vi "Train Track SVM.vi"(8 "error in (no error)":errorcluster, 9 "Classifier File":path=path "C:/Users/Andrew/Documents/Apatite to Zircon Code/Track Finding/TrackClassifier.svm", 10 "Non-track Data File":path=path "C:/Users/Andrew/Documents/Apatite to Zircon Code/Track Finding/Non-track Data.csv", 11 "Track Data File":path=path "C:/Users/Andrew/Documents/Apatite to Zircon Code/Track Finding/Track Data.csv") -> (0 "error out":errorcluster, 1 "Class Predictive Value":dbl[](array[numeric]) format="%.2f", 2 "Classification Distribution":i32[][](array[numeric]), 3 "Accuracy":sgl format="%.2f")   [LabVIEW 2013]
uses:
  <vilib>/vision/Classification.llb/IMAQ SVM Kernel Options.ctl
  <vilib>/vision/Classification.llb/IMAQ SVM Model Options.ctl
  <vilib>/Utility/file.llb/Read From Spreadsheet File (DBL).vi
  <vilib>/vision/NI_Vision_Development_Module.lvlib
panel:
  in  "Model Options":T1={"SVM Model"=enum."C-SVC", "Tolerance"=0.001, "Max. Iteration"=100000, "Nu"=0.1, "Shrinking"=TRUE, "Cost"=1.0, "Weighted Cost"=[]}
  in  "Kernel Options":T2={"Kernel"=enum."Linear", "Degree"=3, "Gamma"=1.0, "Coefficient"=0.0, "Sigma"=1.0, "Cache(MB)"=10.0}
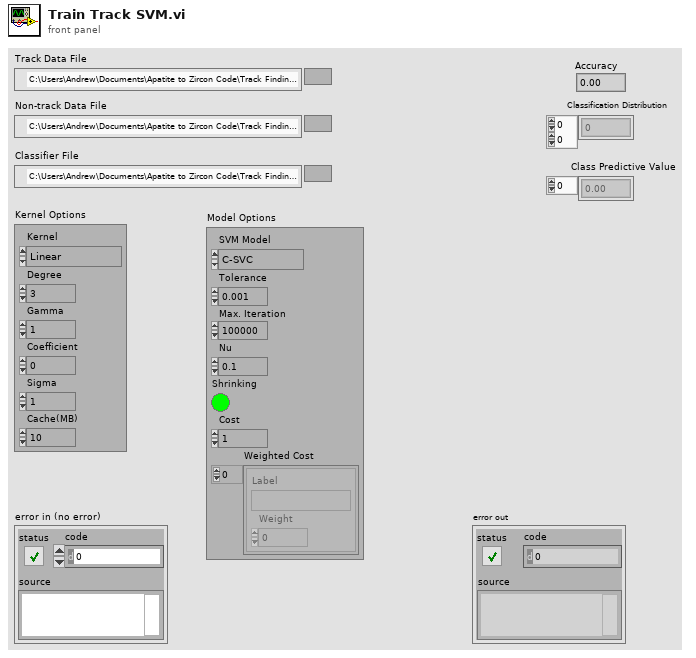
[diagram p1: front panel]
types:
  T1 = typedef "IMAQ SVM Model Options.ctl" = cluster{"SVM Model":enum32{"C-SVC", "nu-SVC", "One Class"}, "Tolerance":dbl, "Max. Iteration":i32, "Nu":dbl, "Shrinking":bool, "Cost":dbl, "Weighted Cost":cluster{"Label":string, "Weight":dbl}[]}
  T2 = typedef "IMAQ SVM Kernel Options.ctl" = cluster{"Kernel":enum32{"Linear", "Polynomial", "Gaussian", "RBF"}, "Degree":i32, "Gamma":dbl, "Coefficient":dbl, "Sigma":dbl, "Cache(MB)":dbl}
  T3 = typedef "Image Type" = u32
  T4 = typedef "IMAQ Image.ctl" = refnum<image>
  T5 = typedef "IMAQ Classifier Session.ctl" = refnum<k1>
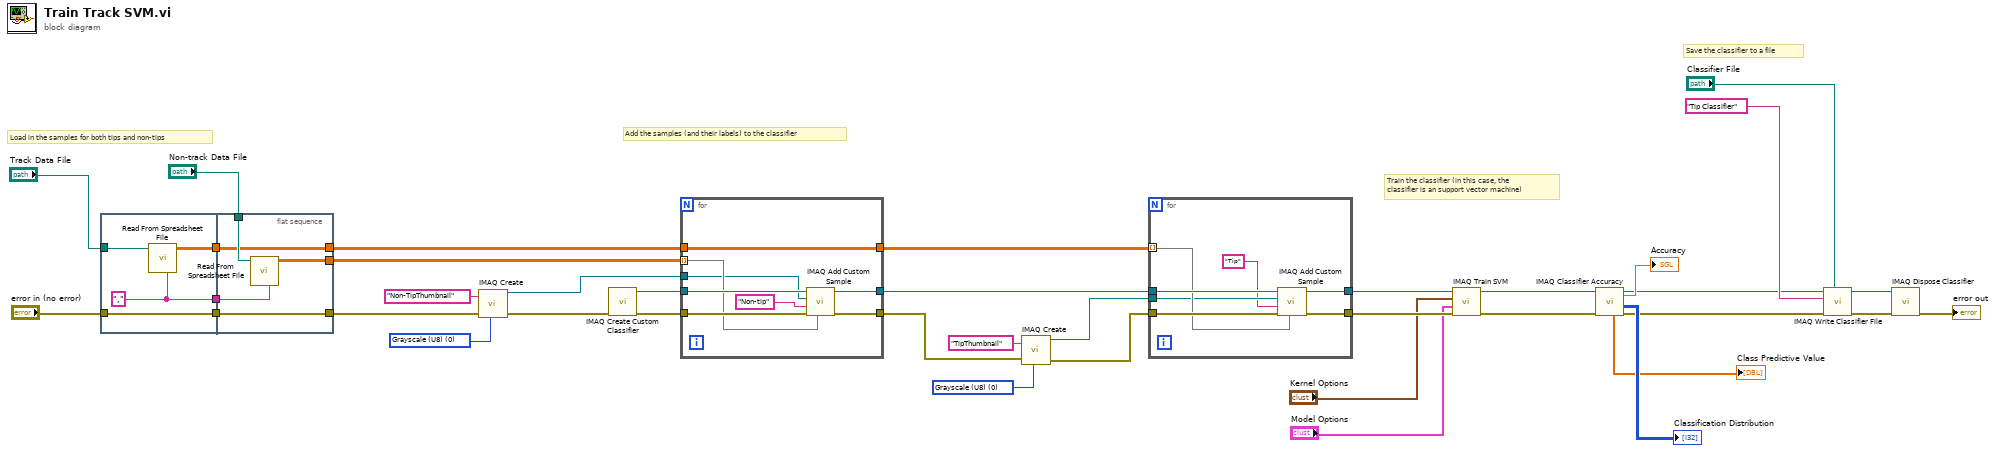
[diagram p0: block diagram]
diagram:
  w27 = T3 0 items=["Grayscale (U8)", "Grayscale (I16)", "Grayscale (SGL)", "Complex (CSG)", "RGB (U32)", "HSL (U32)", "RGB (U64)", "Grayscale (U16)"] ("Image Type")
  w29 = T3 0 items=["Grayscale (U8)", "Grayscale (I16)", "Grayscale (SGL)", "Complex (CSG)", "RGB (U32)", "HSL (U32)", "RGB (U64)", "Grayscale (U16)"] ("Image Type")
  # "Save the classifier to a file"
  # "Train the classifier (in this case, the \nclassifier is an support vector machine)"
  # "Add the samples (and their labels) to the classifier"
  # "Load in the samples for both tips and non-tips"
  n1 = flat-sequence {
    tunnel: "Track Data File" -> [w42]
    tunnel: "error in (no error)" -> [w41]
    tunnel: [w41] -> w36
    tunnel: [w40] -> w34
    tunnel: [w39] -> w22
    tunnel: [w47] -> w25
    tunnel: w36 -> [w47]
    tunnel: "Non-track Data File" -> [w46]
    tunnel: [w45] -> w20
    tunnel: w34 -> [w44]
    tunnel: [w44] -> w21
    tunnel: w22 -> [w43]
    frame #0 {
      w39 = "," ("delimiter (\\t)")
      n2 = call-poly <vilib>:"Read From Spreadsheet File.vi"("delimiter (\\t)"=w39, "file path (dialog if empty)"=w42) -> ("all rows"=w40:dbl[][])  [unwired: 5 in, 4 out]
    }
    frame #1 {
      n3 = call-poly <vilib>:"Read From Spreadsheet File.vi"("delimiter (\\t)"=w43, "file path (dialog if empty)"=w46) -> ("all rows"=w45:dbl[][])  [unwired: 5 in, 4 out]
    }
  }
  n4 = call "IMAQ Create"("Image Name"="Non-TipThumbnail", "Image Type"=w27, "error in (no error)"=w25) -> ("New Image"=w19:T4, "error out"=w18:errorcluster)  [unwired: 2 in]
  n5 = call "IMAQ Create Custom Classifier"("error in (no error)"=w18) -> ("error out"=w32:errorcluster, "Classifier Session"=w33:T5)  [unwired: 9 in]
  n6 = for {
    tunnel: w20 -> [w53] mode=indexing
    tunnel: w33 -> [w54]
    tunnel: w32 -> [w55]
    tunnel: [w52] -> w30
    tunnel: [w51] -> w24
    tunnel: w21 -> [w50]
    tunnel: [w50] -> w31
    tunnel: w19 -> [w48]
    n7 = call "IMAQ Add Custom Sample"("Feature Vector"=w53, "error in (no error)"=w55, "Class"="Non-tip", "Image"=w48, "Classifier Session"=w54) -> ("error out"=w51:errorcluster, "Classifier Session (dup)"=w52:T5)  [unwired: 5 in]
  }
  n8 = call "IMAQ Create"("Image Name"="TipThumbnail", "Image Type"=w29, "error in (no error)"=w24) -> ("New Image"=w17:T4, "error out"=w16:errorcluster)  [unwired: 2 in]
  n9 = for {
    tunnel: w31 -> [w60] mode=indexing
    tunnel: w30 -> [w61]
    tunnel: w16 -> [w62]
    tunnel: [w59] -> w11
    tunnel: [w58] -> w10
    tunnel: w17 -> [w57]
    n10 = call "IMAQ Add Custom Sample"("Feature Vector"=w60, "error in (no error)"=w62, "Class"="Tip", "Image"=w57, "Classifier Session"=w61) -> ("error out"=w58:errorcluster, "Classifier Session (dup)"=w59:T5)  [unwired: 5 in]
  }
  n11 = call "IMAQ Train SVM"("error in (no error)"=w10, "Model Options"="Model Options", "Kernel Options"="Kernel Options", "Classifier Session"=w11) -> ("error out"=w3:errorcluster, "Classifier Session (dup)"=w4:T5)  [unwired: 4 in, 2 out]
  n12 = call "IMAQ Classifier Accuracy"("error in (no error)"=w3, "Classifier Session"=w4) -> ("error out"=w1:errorcluster, "Classification Distribution"=→"Classification Distribution":i32[][], "Classifier Session (dup)"=w2:T5, "Class Predictive Value"=→"Class Predictive Value":dbl[], "Accuracy"=→"Accuracy":sgl)  [unwired: 3 in, 2 out]
  n13 = call "IMAQ Write Classifier File"("File Path"="Classifier File", "error in (no error)"=w1, "Description"="Tip Classifier", "Classifier Session"=w2) -> ("error out"=w15:errorcluster, "Classifier Session (dup)"=w14:T5)  [unwired: 6 in]
  n14 = call "IMAQ Dispose Classifier"("error in (no error)"=w15, "Classifier Session"=w14) -> ("error out"=→"error out":errorcluster)  [unwired: 9 in]
